vi "Get Comparator Tags.vi"(8 "error in (no error)":errorcluster, 11 "TreeControl in":refnum<vi>) -> (0 "error out":errorcluster, 1 "#ofComparators (New ComparatorID)":i32, 2 "Comparator Tags":string[](array[string]), 3 "TreeControl out":refnum<vi>)   [LabVIEW 2018]
uses:
  TypeDefs/Tree Item Type.ctl
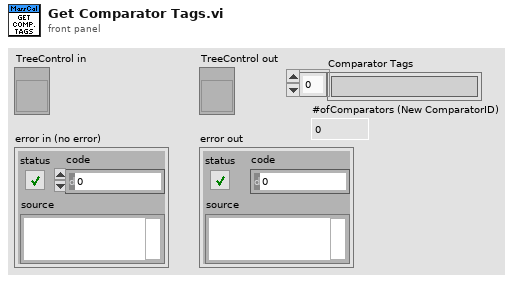
[diagram p1: front panel]
types:
  T1 = typedef "Tree Item Type.ctl" = enum16{"Comparator", "Temp Group", "Press Group", "Hygro Group", "Thermometer", "PressureTransducer", "Hygrometers", "Add Comparator", "Add Thermometer", "Add Barometer", "Add Hygrometer"}
  T2 = typedef "Test Manager Tree Tag.ctl" = cluster{"ItemType":T1, "VISA Resource":refnum<visa-resource-name>, "Name":string, "Channel #":u16, "ComparatorID":u16}
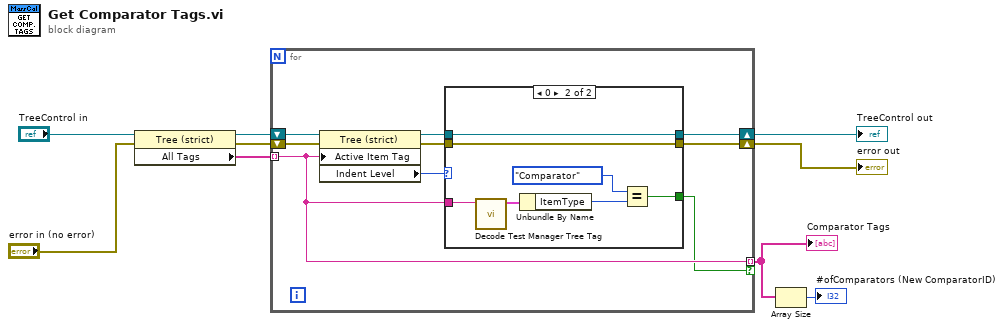
[diagram p0: block diagram]
diagram:
  n1 = property class="Tree (strict)"(reference="TreeControl in", error in="error in (no error)") -> (reference out=w5:refnum<vi>, error out=w7:errorcluster, "All Tags"=w3:string[])
  n2 = for {
    shift-right: [w12] -> w6
    shift-left: w7 -> [w18]
    shift-right: [w13] -> w4
    shift-left: w5 -> [w17]
    tunnel: w3 -> [w11] mode=indexing
    tunnel: [w11] -> w2 mode=indexing if=w10
    n3 = property class="Tree (strict)"(reference=w17, error in=w18, "Active Item Tag"=w11) -> (reference out=w15:refnum<vi>, error out=w14:errorcluster, "Indent Level"=w16:i32)
    n4 = case shown="0" w16 {
      tunnel: w15 -> [w20 w22]
      tunnel: w14 -> [w19 w21]
      tunnel: w11 -> [_ w27]
      tunnel: [_ w23] -> w10
      tunnel: [w20 w22] -> w13
      tunnel: [w19 w21] -> w12
      frame Default {
      }
      frame 0 {
        n5 = call "Decode Test Manager Tree Tag.vi"("Tag"=w27) -> ("Test Manager Tree Tag"=w26:T2)  [unwired: 9 in, 1 out]
        n6 = Unbundle By Name(w26) -> ("ItemType"=w25:T1)
        n7 = Equal?(x=Tree_Item_Type."Comparator", y=w25) -> (x = y?=w23:bool)
      }
    }
  }
  "TreeControl out" <- w4
  "error out" <- w6
  "Comparator Tags" <- w2
  n8 = Array Size(array=w2) -> (size(s)=→"#ofComparators (New ComparatorID)":i32)
